vi "03Foot_GetDelta1.vi"(11 "Array":u8[](array[numeric])) -> (3 "Wave1 Data":i32)   [LabVIEW 2015]
panel:
  # "This VI is a replacement to \"Foot_GetWave\" in such that\nit only acquires the first value from Waveform1"
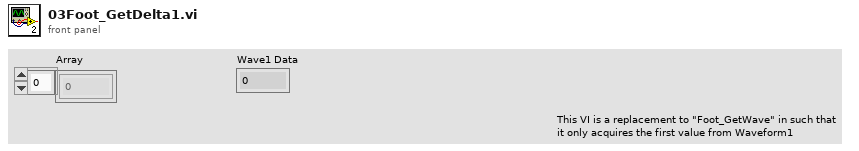
[diagram p1: front panel]
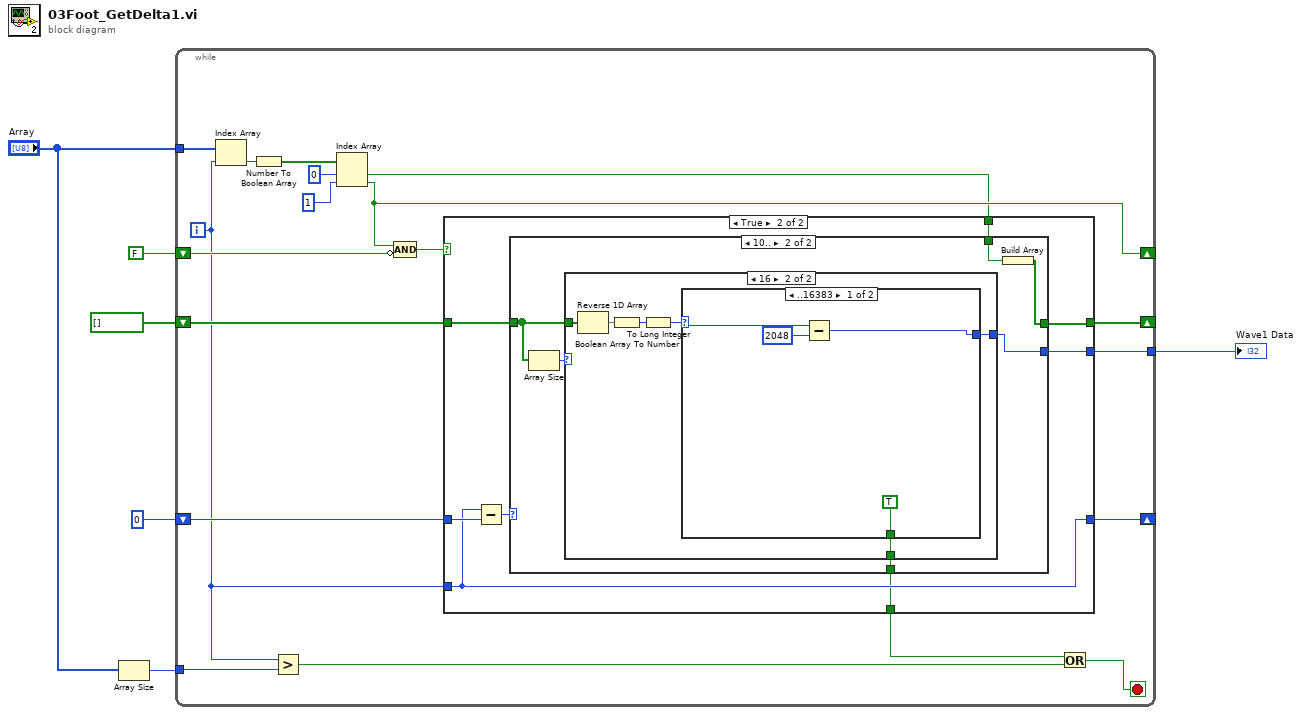
[diagram p0: block diagram]
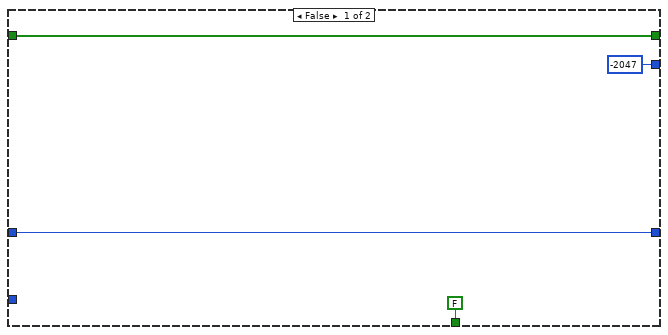
[diagram p2: hidden frame]
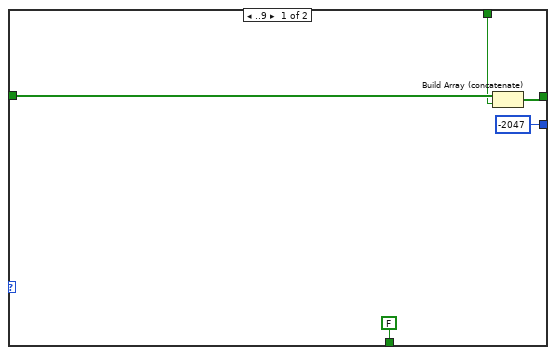
[diagram p3: hidden frame]
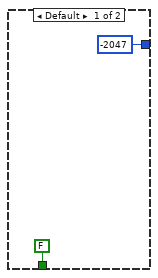
[diagram p4: hidden frame]
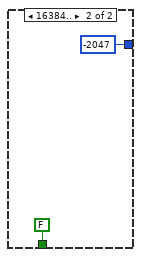
[diagram p5: hidden frame]
diagram:
  n1 = Array Size(array="Array") -> (size(s)=w1:i32)
  n2 = while {
    tunnel: "Array" -> [w14]
    shift-right: [w22] -> _
    shift-left: FALSE -> [w21]
    shift-right: [w18] -> _
    shift-left: 0 -> [w19]
    shift-right: [w16] -> _
    shift-left: bool[] [] -> [w15]
    tunnel: [w12] -> w3
    tunnel: w1 -> [w11]
    i -> [w10]
    stop <- w9 stop-if-true
    n3 = Index Array(array=w14, index=w10) -> (element=w13:u8)
    n4 = Number To Boolean Array(number=w13) -> (Boolean array=w25:bool[])
    n5 = Greater?(x=w10, y=w11) -> (0:w8:bool)
    n6 = Index Array(array=w25, index #1=0 ("index"), index #2=1 ("index")) -> (element #1=w17:bool, element #2=w22:bool)
    n7 = Compound Arithmetic op=AND(w22, invert w21) -> (w20:bool)
    n8 = case shown="True" w20 {
      tunnel: w10 -> [_ w35]
      tunnel: w19 -> [w29 w37]
      tunnel: [w29 w35] -> w18
      tunnel: w17 -> [_ w34]
      tunnel: [w28 w32] -> w16
      tunnel: w15 -> [w28 w33]
      tunnel: [-2047 w31] -> w12
      tunnel: [FALSE w30] -> w7
      frame False {
      }
      frame True {
        n9 = Subtract(x=w35, y=w37) -> (x-y=w36:i32)
        n10 = case shown="10.." w36 {
          tunnel: w34 -> [w41 w47]
          tunnel: w33 -> [w42 w45]
          tunnel: [w40 w48] -> w32
          tunnel: [-2047 w44] -> w31
          tunnel: [FALSE w43] -> w30
          frame ..9 {
            n11 = Build Array (concatenate)(w42, w41) -> (w40:bool[])
          }
          frame 10.. {
            n12 = Array Size(array=w45) -> (size(s)=w46:i32)
            n13 = case shown="16" w46 {
              tunnel: w45 -> [_ w56]
              tunnel: [-2047 w52] -> w44
              tunnel: [FALSE w51] -> w43
              frame Default {
              }
              frame 16 {
                n14 = Reverse 1D Array(array=w56) -> (reversed array=w55:bool[])
                n15 = Boolean Array To Number(Boolean array=w55) -> (number=w54:u32)
                n16 = To Long Integer(number=w54) -> (32bit integer=w53:i32)
                n17 = case shown="..16383" w53 {
                  selector: w53 -> [w60 _]
                  tunnel: [w58 -2047] -> w52
                  tunnel: [TRUE FALSE] -> w51
                  frame ..16383 {
                    n18 = Subtract(x=w60, y=2048) -> (x-y=w58:i32)
                  }
                  frame 16384.. {
                  }
                }
              }
            }
            n19 = Build Array(w47) -> (w48:bool[])
          }
        }
      }
    }
    n20 = Or(x=w7, y=w8) -> (x .or. y?=w9:bool)
  }
  "Wave1 Data" <- w3
